vi "slicevisualizerfromstack.vi"() -> ()   [LabVIEW 2017]
panel:
  in  "Enum":enum16{"X", "Y", "Z", ""}(ring)
  in  "index":i32(slide)=210 scale=0.0..512.0
  in  "stop":bool
  out "Image":T1(plugin-control)
  in  "Experiment folder path":path
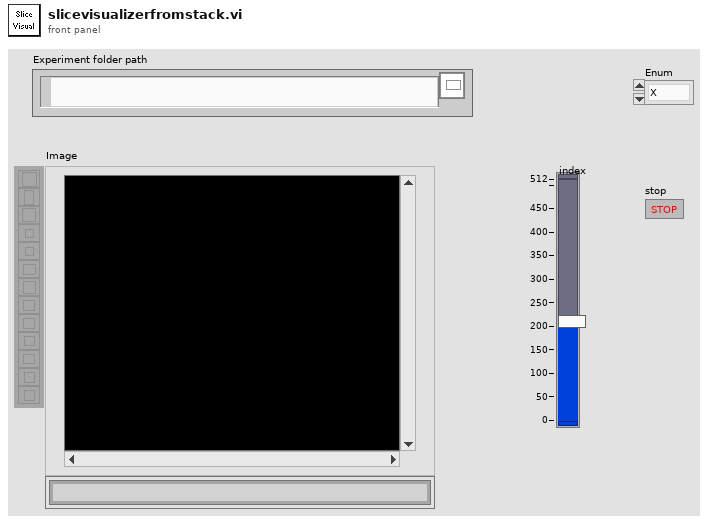
[diagram p1: front panel]
types:
  T1 = typedef "IMAQ Image.ctl" = refnum<image>
  T2 = typedef "Image Type" = u32
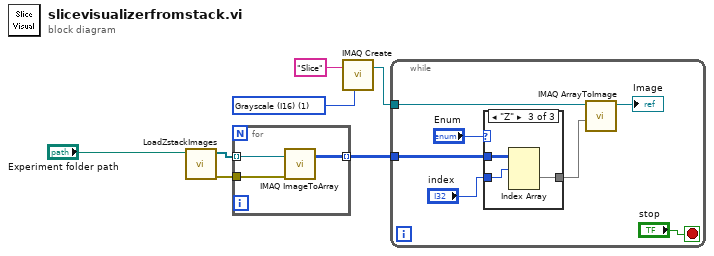
[diagram p0: block diagram]
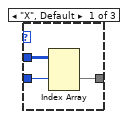
[diagram p2: hidden frame]
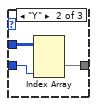
[diagram p3: hidden frame]
diagram:
  w1 = T2 1 items=["Grayscale (U8)", "Grayscale (I16)", "Grayscale (SGL)", "Complex (CSG)", "RGB (U32)", "HSL (U32)", "RGB (U64)", "Grayscale (U16)"] ("Image Type")
  n1 = call "LoadZstackImages.vi"("Experiment folder path"="Experiment folder path") -> ("Error Out"=w4:errorcluster, "RedImageArray"=w6:T1[])  [unwired: 3 in, 6 out]
  n2 = for {
    tunnel: w6 -> [w10] mode=indexing
    tunnel: [w9] -> w5 mode=indexing
    tunnel: w4 -> [w8]
    n3 = call "IMAQ ImageToArray"("error in (no error)"=w8, "Image"=w10) -> ("Image Pixels (I16)"=w9:i16[][])  [unwired: 2 in, 4 out]
  }
  n4 = call "IMAQ Create"("Image Name"="Slice", "Image Type"=w1) -> ("New Image"=w3:T1)  [unwired: 3 in, 1 out]
  n5 = while {
    tunnel: w5 -> [w17]
    tunnel: w3 -> [w11]
    stop <- "stop" stop-if-true
    n6 = case shown="\"Z\"" "Enum" {
      tunnel: w17 -> [w20 w23 w26]
      tunnel: [w18 w22 w25] -> w16
      tunnel: "index" -> [w19 w21 w24]
      frame "X", Default {
        n7 = Index Array(array=w20, index (dim 1)=w19) -> (element=w18:i16[][])  [unwired: 2 in]
      }
      frame "Y" {
        n8 = Index Array(array=w23, index (dim 2)=w21) -> (element=w22:i16[][])  [unwired: 2 in]
      }
      frame "Z" {
        n9 = Index Array(array=w26, index (dim 0)=w24) -> (element=w25:i16[][])  [unwired: 2 in]
      }
    }
    n10 = call "IMAQ ArrayToImage"("Image Pixels (I16)"=w16, "Image"=w11) -> ("Image Out"=→"Image":T1)  [unwired: 8 in, 1 out]
  }
